vi "Action Define Instrument Name.vi"(0 "VISA resource name":refnum<visa-resource-name>, 5 "Logical Instrument Name":string, 7 "Logical Instrument Number":u32, 11 "error in (no error)":errorcluster) -> (4 "VISA resource name out":refnum<visa-resource-name>, 15 "error out":errorcluster)   [LabVIEW 2012, in "NH Research Regenerative Test Series.lvlib"]
doc: "Sets the <B>Logical Instrument Name</B> and associates it with a logical instrument number, <B>Logical Instrument Number</B>. There can only be one logical instrument name associated with a given instrument number.\n\nNOTE: The 4900 only has one logical instrument so the only valid instrument number is 1."
uses:
  <instrlib>/NH Research Regenerative Test Series/NH Research Regenerative Test Series.lvlib
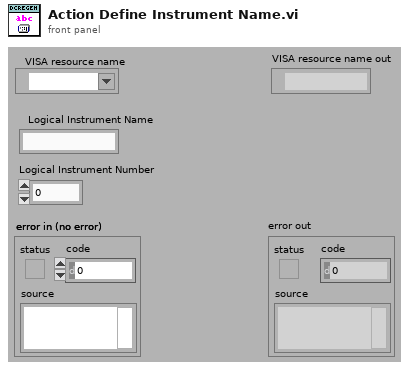
[diagram p1: front panel]
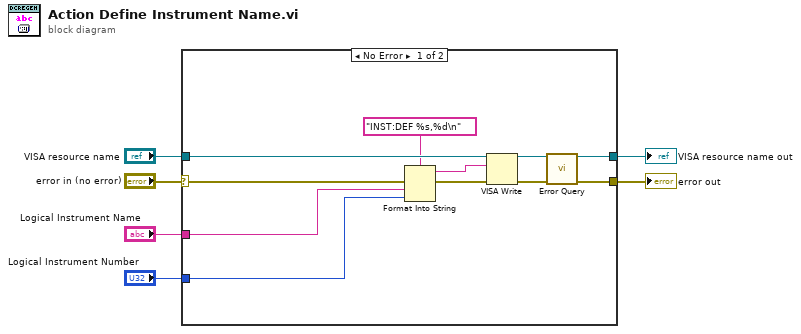
[diagram p0: block diagram]
diagram:
  n1 = case shown="No Error" "error in (no error)" {
    selector: "error in (no error)" -> [w12 w19]
    tunnel: "VISA resource name" -> [w17 w18]
    tunnel: [w14 w18] -> w5
    tunnel: [w13 w19] -> w4
    tunnel: "Logical Instrument Name" -> [w8 _]
    tunnel: "Logical Instrument Number" -> [w7 _]
    frame No Error {
      n2 = Format Into String(format string="INST:DEF %s,%d\n" ("Command"), error in=w12, w8, w7) -> (resulting string=w15:string, error out=w11:errorcluster)  [unwired: 1 in]
      n3 = VISA Write(VISA resource name=w17, write buffer=w15, error in (no error)=w11) -> (VISA resource name out=w10:refnum<visa-resource-name>, error out=w9:errorcluster)  [unwired: 1 out]
      n4 = call <instrlib>:"Error Query.vi"("VISA resource name"=w10, "error in (no error)"=w9) -> ("VISA resource name out"=w14:refnum<visa-resource-name>, "error out"=w13:errorcluster)  [unwired: 10 in, 2 out]
    }
    frame Error {
    }
  }
  "error out" <- w4
  "VISA resource name out" <- w5
